vi "Assemble.vi"() -> ()   [LabVIEW 2015]
uses:
  Downloads/fpga_modify-default-myrio-personality/Sub VIs/Utilities/Start Boolean.ctl
  <vilib>/Platform/TimedLoop/XDataNode/timing_clust.ctl
  <vilib>/Platform/TimedLoop/XDataNode/nitl_modes.ctl
  <vilib>/Platform/TimedLoop/XDataNode/wakeup.ctl
  <vilib>/rvi/Emulation/niFpgaGetClockAttributes.vi
  <vilib>/rvi/Emulation/niFpgaSctlEmulationGetInTimedLoop.vi
  <vilib>/rvi/Emulation/niFpgaEmulationReportErrorSimple.vi
  <vilib>/rvi/eio/common/nirviEmuTemplateMethod_errors.vi
  <vilib>/rvi/Emulation/niFpgaCriticalErrorInLSC.vi
  <vilib>/rvi/Emulation/niFpgaProcessEmulError.vi
  <vilib>/rvi/Emulation/niFpgaEmulationIsFPGAContextNoSignature.vi
  <vilib>/rvi/errors/niFpgaSetErrorForExecOnDevCompSimple.vi
  <vilib>/rvi/eio/common/nirviEmuReportErrorAndStop.vi
  <vilib>/rvi/DataTransferAndStorage/Container/Common/niFpgaContainerGetUniqueNameForEmu.vi
  <vilib>/rvi/FIFO/Fifo_Resource/nirvififoEmulationSetSize.vi
  <vilib>/rvi/FIFO/Fifo_Resource/nirviFifoEmulationQueueMgr.vi
  <instcachedir>/0/nirviFifoEmulationQueueMgr_E5CAEC123FF24DC58D834DCA3CDAA9B5.lvgen/nirviFifoEmulationQueueMgr_E5CAEC123FF24DC58D834DCA3CDAA9B5_002.vi
  <vilib>/rvi/FIFO/Fifo_Resource/nirvififoEmulationDetermineInputValidOut.vi
  <vilib>/rvi/FIFO/Fifo_Resource/nirvififoEmulationCreateLock.vi
  <vilib>/rvi/FIFO/Fifo_Resource/nirvififoEmulationObtainLock.vi
  <vilib>/rvi/FIFO/Fifo_Resource/nirvififoEmulationReleaseLock.vi
  <vilib>/rvi/occurrence/nirviWaitOnOccurrenceBase.vi
  <vilib>/rvi/errors/nirviReportUnexpectedCaseInternalError.vi
  <vilib>/rvi/errors/nirviReportUnexpectedCaseInternalError (U32).vi
  <vilib>/Utility/error.llb/Clear Errors.vi
  <vilib>/rvi/DataTransferAndStorage/Container/Common/niFpgaContainerSetEmuInfo.vi
  <vilib>/eio/EIONode/EIONode.xnode
  <vilib>/rvi/DataTransferAndStorage/Container/XNode/niFpgaContainer.xnode
  <vilib>/rvi/FIFO/Fifo_Resource/nirvififoEmulationWrite.vi
  <vilib>/rvi/FIFO/Fifo_Resource/nirvififoEmulationRead.vi
  <vilib>/Platform/TimedLoop/XDataNode/XDataNode.xnode
  <vilib>/rvi/LocalResourceManager/LocalResourceManager.xnode
  <vilib>/rvi/Arithmetic/AddSubMult/XNode/nirviSatArithmetic.xnode
  <vilib>/Platform/TimedLoop/XDataNode/XDNodeRunTimeDep.lvlib
panel:
  out "time of flight 4":u32
  out "time of flight 3":u32
  out "time of flight 2":u32
  out "time of flight 1":u32
  in  "Trigger pulse interval 4":u32=200
  in  "Trigger pulse interval 3":u32=200
  in  "Trigger pulse interva 2":u32=200
  out "Velocity (Counts/Interval) 4":i32
  out "Acceleration (Counts/Interval) 4":i32
  in  "Velocity Interval (uSec) 4":u32=1000
  out "Velocity (Counts/Interval) 3":i32
  out "Acceleration (Counts/Interval) 3":i32
  in  "Velocity Interval (uSec) 3":u32=1000
  out "Velocity (Counts/Interval) 2":i32
  out "Acceleration (Counts/Interval) 2":i32
  in  "Velocity Interval (uSec) 2":u32=1000
  out "Velocity (Counts/Interval)":i32
  out "Acceleration (Counts/Interval)":i32
  in  "Velocity Interval (uSec)":u32=1000
  out "Position 4":i32
  in  "Position Reset 4":bool
  out "Position 3":i32
  in  "Position Reset 3":bool
  in  "En8":bool
  in  "En7":bool
  in  "En6":bool
  in  "En5":bool
  in  "En4":bool
  in  "En3":bool
  in  "En2":bool
  in  "En1":bool
  in  "Relay Motor 1":bool=TRUE
  in  "Relay motor 2":bool=TRUE
  in  "Relay motor 3":bool=TRUE
  in  "Relay motor 4":bool=TRUE
  in  "Relay kebocoran":bool=TRUE
  in  "tof 8":u32=200
  in  "EI8":bool=TRUE
  in  "ton 8":u32=10
  in  "E8O":bool=TRUE
  in  "tof 7":u32=200
  in  "EI7":bool=TRUE
  in  "ton 7":u32=10
  in  "E7O":bool=TRUE
  in  "tof 6":u32=200
  in  "EI6":bool=TRUE
  in  "ton 6":u32=10
  in  "E6O":bool=TRUE
  in  "tof 5":u32=200
  in  "EI54":bool=TRUE
  in  "ton 5":u32=10
  in  "E5O":bool=TRUE
  in  "tof 4":u32=200
  in  "EI4":bool=TRUE
  in  "ton 4":u32=10
  in  "E4O":bool=TRUE
  in  "tof 3":u32=200
  in  "EI3":bool=TRUE
  in  "ton 3":u32=10
  in  "E3O":bool=TRUE
  in  "tof 2":u32=200
  in  "ton 2":u32=10
  in  "EI2":bool=TRUE
  in  "EI1":bool=TRUE
  in  "E2O":bool=TRUE
  in  "E1O":bool=TRUE
  in  "ton":u32=10
  in  "tof":u32=200
  out "Position 2":i32
  in  "Position Reset 2":bool
  in  "Position Reset":bool
  out "Position 1":i32
  in  "I2C.A.DATO 2":u8
  out "I2C.A.DATI 2":u8
  in  "I2C.A.ADDR 2":u8 format="%08.0f"
  in  "I2C.A.CNTR 2":u8=213
  in  "I2C.A.CNTL 2":u8 format="%08b"
  out "I2C.A.STAT 2":u8 format="%08b"
  in  "I2C.A.CNFG 2":u8=1 format="%08b"
  in  "Execute?":T1
  in  "OUT 0":bool
  out "LIMIT BAWAH":bool
  out "LIMIT ATAS":bool
  out "BUTTON":bool
  in  "Trigger pulse interval 1":u32=200
  out "Channel 1":u32
  out "Channel) 2":u32
  out "Channel 3":u32
  in  "IRQ.TIMER.SETTIME":T1
  in  "IRQ.TIMER.WRITE":u32
  out "IRQ.TIMER.READ":u32
  out "ACC.Z.VAL":u16
  out "SYS.ACC.RDY":bool
  out "ACC.Y.VAL":u16
  out "ACC.X.VAL":u16
  in  "DO.LED3:0":u8 format="%04b"
  out "DI.BTN":u8 format="%08b"
  in  "IRQ.DI_BTN.ENA":bool
  in  "IRQ.DI_BTN.RISE":bool
  in  "IRQ.DI_BTN.FALL":bool
  in  "IRQ.DI_BTN.CNT":u32
  in  "IRQ.DI_BTN.NO":u8
  out "SYS.RDY":bool
  out "AI.A_0.VAL":u16
  out "V sensor":u16
  out "Water_LVL1":u16
  out "Water_LVL2":u16
  out "ACS712(1)":u16
  out "ACS712(2)":u16
  out "ACS712(3)":u16
  out "ACS712(4)":u16
  out "SYS.AI.RDY":bool
  out "AI.AudioIn_L.VAL":u16
  out "AI.AudioIn_R.VAL":u16
  out "AI.C_1.VAL":u16
  out "AI.C_0.VAL":u16
  in  "IRQ.AI_A_3:0.CNFG":u8 format="%.0b"
  in  "IRQ.AI_A_0.THRESHOLD":u16
  in  "IRQ.AI_A_1.THRESHOLD":u16
  in  "IRQ.AI_A_0.NO":u8
  in  "IRQ.AI_A_1.NO":u8
  in  "IRQ.AI_A_1.HYSTERESIS":u16=17
  in  "IRQ.AI_A_0.HYSTERESIS":u16=17
  in  "AO.A_0.VAL":u16
  in  "AO.A_1.VAL":u16
  in  "AO.B_0.VAL":u16
  in  "AO.B_1.VAL":u16
  in  "AO.AudioOut_L.VAL":u16
  in  "AO.AudioOut_R.VAL":u16
  in  "AO.SYS.GO":T1
  in  "AO.C_1.VAL":u16
  in  "AO.C_0.VAL":u16
  out "AO.SYS.STAT":bool
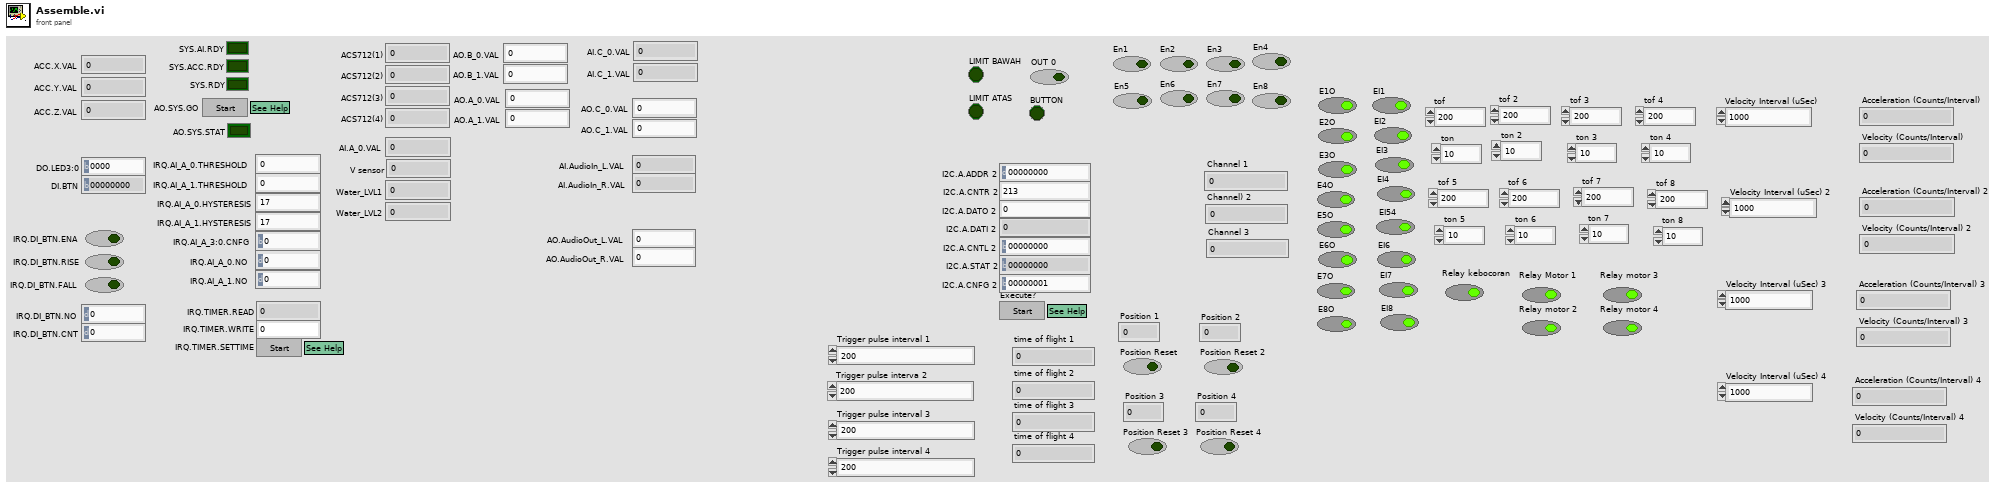
[diagram p1: front panel]
types:
  T1 = typedef "Start Boolean.ctl" = bool
  T2 = typedef "XDNodeRunTimeDep.lvlib/timing_clust.ctl" = cluster{"Expected End [f-1]":u64, "Actual End [f-1]":u64, "Finished Late? [f-1]":bool, "Expected End [i-1]":u64, "Actual End [i-1]":u64, "Finished Late? [i-1]":bool, "Expected Start [i]":u64, "Actual Start [i]":u64, "Expected Start [f]":u64, "Actual Start [f]":u64, "Source Name":string, "Structure Name":string, "Period":i64, "Deadline":i64, "Offset":i64, "Start":i64, "Priority":i32, "Timeout":i32, "Mode":T3, "Wakeup Reason":T4, "Error":errorcluster, "Source Type":string, "Secondary Source Type":string, "Global End Time":u64, "Global Start Time":u64, "Frame Duration":u64, "Iteration Duration":u64, "Assigned CPU":i32, "I/O Scan Engine Mode":u32}
  T3 = typedef "XDNodeRunTimeDep.lvlib/nitl_modes.ctl" = enum32{"No Change", "Process missed periods, maintain original phase", "Discard missed periods, maintain original phase", "Process missed periods, ignore original phase", "Discard missed periods, ignore original phase"}
  T4 = typedef "XDNodeRunTimeDep.lvlib/wakeup.ctl" = enum32{"Normal", "Aborted", "Asynchronous wakeup", "Timing source error", "Timed loop error", "Timeout"}
diagram:
  # "The Timed Loop does not allow writing the same FIFO outside the Timed Loop. Use another FIFO to push all interrupts from Button in the Timed Loop to the IRQ Queue."
  # "The accelerometer nodes take some time before the FPGA can first read the values. This is because it takes time to read from the accelerometer. An iteration of the While Loop will not complete until the accelerometer values have been read.\n\nAfter the completion of the first iteration of the While Loop, all indicators have valid values."
  # "The analog output nodes take some time before the FPGA write the values to the pins. The GO and STAT registers are used to handshake between the FPGA and host. When the host wants the values to be written, the host sets the GO register to TRUE. If the host reads the STAT register before setting the value of the GO register, it can wait for the value of the STAT register to invert. The value inversion tells the host that the output values have been written."
  # "The analog input nodes take some time before the FPGA can first read the values. This is because it takes time to set up the Analog-to-Digital converter (ADC) and convert the first reading. An iteration of the While Loop will not complete until all the analog input channels have been sampled.\n\nAfter the completion of the first iteration of the While Loop, all indicators have valid values."
  # "Note: On some hardware a \"ghosting effect\" may occur on any unconnected AI channels. For example, if channel AI0 is connected and channels AI1~AI7 are not connected the the value read at AI0 may be seen on indicators AI1~AI7. This is common for hardware that use a multiplexed (MUXed) Analog-to-Digital converter (ADC), because the input analog signal is used to charge a capacitor which does not discharge before the unconnected channel is read.\n\nYou can hide the \"ghosting effect\" by using an mask register. This register is used to decide when the indicator should be updated."
  # "The FPGA timer fires the interrupt request (IRQ) when TIMER.Read counts down to zero. If TIMER.Read is not zero, it counts down to one per microsecond."
  # "The only interface that sends interrupts to the RT side. Timer interrupts, analog input interrupts, digital input interrupts, and SPI interrupt share this interface.\n\nAll interrupts work in sequence. One interrupt waits until the previous interrupt request (IRQ) gets acknowledged on the RT side."
  # "NOTE: The SYS.RDY Boolean MUST exist and must become TRUE at some point. Otherwise, the myRIO VIs will not function correctly."
  # "There is some delay between the time when the FPGA code starts and the time when the analog inputs, accelerometer, and scaling values outputs are valid. If the host wants to ensure that there are valid values in theses registers it should wait for each subsystem to finish its initialization process. \n\nWhen all subsystems have finished initializinig, the SYS.RDY indicator turns true. The host can poll the SYS.RDY indicator to determine the status of the FPGA. Alternatively, the host can poll the individual SYS.xx.RDY indicators to determine the status of the individual subsystems.\n\nThis loop continues indefinitely, essentially making SYS.RDY a read-only register."
  n1 = while {
    stop <- FALSE stop-if-true
    # "Host Synchronization"
    n2 = local read "SYS.ACC.RDY"() -> (w24:bool)
    n3 = local read "SYS.AI.RDY"() -> (w26:bool)
    n4 = Compound Arithmetic op=AND(w26, w24) -> (→"SYS.RDY":bool)
  }
  n5 = while {
    stop <- FALSE stop-if-true
    # "Interrupt to RT"
    n6 = xnode ("FIFO Method Node")("Timeout"=-1) -> ("Element"=w29:u8)  [unwired: 1 in, 2 out]
    n7 = call <vilib>:"niFPGA Interrupt.vi"("Wait Until Cleared (F)"=TRUE, "IRQ Number (0)"=w29) -> ()  [unwired: 1 in]
  }
  n8 = while {
    stop <- FALSE stop-if-true
    # "Timer"
    n9 = local read "IRQ.TIMER.READ"() -> (w34:u32)
    n10 = Select(t="IRQ.TIMER.WRITE", s="IRQ.TIMER.SETTIME", f=w34) -> (s? t:f=w32:u32)
    n11 = case shown="Default" w32 {
      selector: w32 -> [w38 w41]
      tunnel: [w38 w39] -> w31
      frame 0 {
      }
      frame Default {
        n12 = Decrement(x=w41) -> (x-1=w40:u32)
        n13 = case shown="0" w40 {
          selector: w40 -> [w42 w45]
          tunnel: [w42 w45] -> w39
          frame Default {
          }
          frame 0 {
            w44 = u8 0  # Reserved for Timer IRQ
            n14 = xnode ("FIFO Method Node")("Element"=w44, "Timeout"=-1) -> ()  [unwired: 1 in, 2 out]
          }
        }
      }
    }
    "IRQ.TIMER.READ" <- w31
    n15 = call "Loop Timer"("Count(uSec)"=u8 1 ("Count(mSec)")) -> ()  [unwired: 1 out]
  }
  n16 = xnode "VI-Defined FIFO Configuration"() -> ("FIFO Out"=w20:refnum<k21>)
  n17 = while {
    tunnel: w20 -> [w47]
    i -> [w74]
    stop <- FALSE stop-if-true
    # "Analog Input"
    n18 = xnode "FPGA I/O Node"() -> ("ConnectorA/AI0"=w52:u16, "ConnectorA/AI1"=w51:u16, "ConnectorA/AI2"=→"Water_LVL1":u16, "ConnectorA/AI3"=→"Water_LVL2":u16, "ConnectorB/AI0"=→"ACS712(1)":u16, "ConnectorB/AI1"=→"ACS712(2)":u16, "ConnectorB/AI2"=→"ACS712(3)":u16, "ConnectorB/AI3"=→"ACS712(4)":u16, "ConnectorC/AI0"=w68:i16, "ConnectorC/AI1"=w67:i16, "AudioIn/Left"=w66:i16, "AudioIn/Right"=w65:i16)  [unwired: 12 in, 12 out]
    "AI.A_0.VAL" <- w52
    "V sensor" <- w51
    n19 = Greater Than 0?(x=w74) -> (x > 0?=→"SYS.AI.RDY":bool)
    n20 = Number To Boolean Array(number="IRQ.AI_A_3:0.CNFG") -> (Boolean array=w62:bool[])
    n21 = Index Array(array=w62) -> (element #1=w60:bool, element #2=w59:bool, element #3=w57:bool, element #4=w56:bool)  [unwired: 4 in]
    n22 = To Unsigned Word Integer(number=w68) -> (unsigned 16bit integer=→"AI.C_0.VAL":u16)
    n23 = To Unsigned Word Integer(number=w67) -> (unsigned 16bit integer=→"AI.C_1.VAL":u16)
    n24 = To Unsigned Word Integer(number=w66) -> (unsigned 16bit integer=→"AI.AudioIn_L.VAL":u16)
    n25 = To Unsigned Word Integer(number=w65) -> (unsigned 16bit integer=→"AI.AudioIn_R.VAL":u16)
    n26 = call "Check AI IRQ.vi"("Hysteresis"="IRQ.AI_A_1.HYSTERESIS", "FIFO In"=w47, "IRQ Number"="IRQ.AI_A_1.NO", "Threshold"="IRQ.AI_A_1.THRESHOLD", "Analog Value"=w51, "Rising Edge?"=w56, "Enable Interrupt?"=w57) -> ()  [unwired: 5 in]
    n27 = call "Check AI IRQ.vi"("Hysteresis"="IRQ.AI_A_0.HYSTERESIS", "FIFO In"=w47, "IRQ Number"="IRQ.AI_A_0.NO", "Threshold"="IRQ.AI_A_0.THRESHOLD", "Analog Value"=w52, "Rising Edge?"=w59, "Enable Interrupt?"=w60) -> ()  [unwired: 5 in]
  }
  n28 = while {
    stop <- FALSE stop-if-true
    # "Analog Output"
    n29 = feedback #1(FALSE) -> (w80:bool)
    n30 = case shown="True" "AO.SYS.GO" {
      tunnel: "AO.C_0.VAL" -> [_ w102]
      tunnel: "AO.C_1.VAL" -> [_ w101]
      tunnel: "AO.A_0.VAL" -> [_ w106]
      tunnel: "AO.A_1.VAL" -> [_ w105]
      tunnel: "AO.B_0.VAL" -> [_ w104]
      tunnel: "AO.B_1.VAL" -> [_ w103]
      tunnel: "AO.AudioOut_L.VAL" -> [_ w98]
      tunnel: "AO.AudioOut_R.VAL" -> [_ w97]
      tunnel: w80 -> [w91 w94]
      tunnel: [w91 w92] -> w78
      frame False {
      }
      frame True {
        n31 = To Word Integer(number=w102) -> (16bit integer=w100:i16)
        n32 = To Word Integer(number=w101) -> (16bit integer=w99:i16)
        n33 = To Word Integer(number=w98) -> (16bit integer=w96:i16)
        n34 = To Word Integer(number=w97) -> (16bit integer=w95:i16)
        n35 = flat-sequence {
          tunnel: w106 -> [w115]
          tunnel: w105 -> [w114]
          tunnel: w104 -> [w113]
          tunnel: w103 -> [w112]
          tunnel: w100 -> [w111]
          tunnel: w99 -> [w110]
          tunnel: w96 -> [w109]
          tunnel: w95 -> [w108]
          tunnel: w94 -> [w107]
          tunnel: [w107] -> w93
          tunnel: w93 -> [w117]
          tunnel: [w116] -> w92
          frame #0 {
            n36 = xnode "FPGA I/O Node"("ConnectorA/AO0"=w115, "ConnectorA/AO1"=w114, "ConnectorB/AO0"=w113, "ConnectorB/AO1"=w112, "ConnectorC/AO0"=w111, "ConnectorC/AO1"=w110, "AudioOut/Left"=w109, "AudioOut/Right"=w108) -> ()  [unwired: 8 in, 8 out]
          }
          frame #1 {
            n37 = Not(x=w117) -> (.not. x?=w116:bool)
          }
        }
      }
    }
    "AO.SYS.STAT" <- w78
    n38 = feedback-in #1(w78) -> ()
  }
  n39 = while {
    i -> [w122]
    stop <- FALSE stop-if-true
    # "Onboard Accelerometer"
    n40 = xnode "FPGA I/O Node"() -> ("AccelerationX"=w125:i16, "AccelerationY"=w124:i16, "AccelerationZ"=w123:i16)  [unwired: 3 in, 3 out]
    n41 = Greater Than 0?(x=w122) -> (x > 0?=→"SYS.ACC.RDY":bool)
    n42 = To Unsigned Word Integer(number=w125) -> (unsigned 16bit integer=→"ACC.X.VAL":u16)
    n43 = To Unsigned Word Integer(number=w124) -> (unsigned 16bit integer=→"ACC.Y.VAL":u16)
    n44 = To Unsigned Word Integer(number=w123) -> (unsigned 16bit integer=→"ACC.Z.VAL":u16)
  }
  n45 = xnode "VI-Defined FIFO Configuration"() -> ("FIFO Out"=w19:refnum<k21>)
  n46 = node-c288() -> (w22:T2)  [unwired: 1 in]
  n47 = timed-loop {
    timing: w22 -> [_]
    timing-out: [_] -> w21
    tunnel: w19 -> [w129]
    stop <- _ stop-if-true
    # "Onboard DIO"
    n48 = xnode "FPGA I/O Node"() -> ("Button0"=w133:bool)  [unwired: 1 in, 1 out]
    n49 = Number To Boolean Array(number="DO.LED3:0") -> (Boolean array=w138:bool[])
    n50 = Build Array(w133) -> (w141:bool[])
    n51 = Index Array(array=w138) -> (element #1=w137:bool, element #2=w136:bool, element #3=w135:bool, element #4=w134:bool)  [unwired: 4 in]
    n52 = call "DIO IRQ 1-bit.vi"("IRQ.NO"="IRQ.DI_BTN.NO", "IRQ.CNT"="IRQ.DI_BTN.CNT", "FIFO in"=w129, "IRQ.FALL"="IRQ.DI_BTN.FALL", "IRQ.RISE"="IRQ.DI_BTN.RISE", "IRQ.ENA"="IRQ.DI_BTN.ENA", "DIO"=w133) -> ()  [unwired: 5 in]
    n53 = Boolean Array To Number(Boolean array=w141) -> (number=→"DI.BTN":u8)
    n54 = xnode "FPGA I/O Node"("LED0"=w137, "LED1"=w136, "LED2"=w135, "LED3"=w134) -> ()  [unwired: 4 in, 4 out]
  }
  n55 = while {
    stop <- FALSE stop-if-true
    # "Button SCTL Interrupt Buffer"
    n56 = feedback #2(u8 0 ("Element")) -> (w146:u8)
    n57 = feedback #3(FALSE ("Timed Out?")) -> (w150:bool)
    n58 = case shown="False" w150 {
      tunnel: [w152 w154] -> w147
      tunnel: w146 -> [_ w154]
      frame False {
        n59 = xnode ("FIFO Method Node")("Timeout"=-1) -> ("Element"=w152:u8)  [unwired: 1 in, 2 out]
      }
      frame True {
      }
    }
    n60 = feedback-in #2(w147) -> ()
    n61 = xnode ("FIFO Method Node")("Element"=w147, "Timeout"=0) -> ("Timed Out?"=w148:bool)  [unwired: 1 in, 1 out]
    n62 = feedback-in #3(w148) -> ()
  }
  n63 = node-c288(w21) -> ()
  n64 = node-c288() -> (w16:T2)  [unwired: 1 in]
  n65 = timed-loop {
    timing: w16 -> [_]
    timing-out: [_] -> w15
    stop <- _ stop-if-true
    # "Connector ALL DIO"
    n66 = disable-structure shown="Disabled" {
      frame Disabled {
        # "DIGITAL BUTTON LAMP"
        # "LIMIT"
        # "I2C MASTER"
        n67 = call "DIO 1-bit.vi"("DIR"=FALSE, "DIO Refnum"=refnum<k21> "ConnectorB/DIO15") -> ("IN"=→"LIMIT ATAS":bool)  [unwired: 9 in]
        n68 = call "DIO 1-bit.vi"("DIR"=FALSE, "DIO Refnum"=refnum<k21> "ConnectorB/DIO14") -> ("IN"=→"LIMIT BAWAH":bool)  [unwired: 9 in]
        n69 = call "DIO 1-bit.vi"("DIR"=TRUE, "OUT"="OUT 0", "DIO Refnum"=refnum<k21> "ConnectorB/DIO15") -> ()  [unwired: 8 in, 1 out]
        n70 = call "DIO 1-bit.vi"("DIR"=FALSE, "DIO Refnum"=refnum<k21> "ConnectorB/DIO14") -> ("IN"=w156:bool)  [unwired: 9 in]
        n71 = call "DIO_I2C.vi"("I2C.CNFG"="I2C.A.CNFG 2", "I2C.CNTL"="I2C.A.CNTL 2", "I2C.ADDR"="I2C.A.ADDR 2", "I2C.DATO"="I2C.A.DATO 2", "DIO.1/I2C.SDA"=refnum<k21> "ConnectorA/DIO15" ("DIO.1/I2C.SCL"), "I2C.CNTR"="I2C.A.CNTR 2", "DIO.0/I2C.SCL"=refnum<k21> "ConnectorA/DIO14" ("DIO.0/I2C.SDA"), "Execute?"="Execute?", "SELECT"=TRUE) -> ("I2C.DATI"=→"I2C.A.DATI 2":u8, "I2C.STAT"=→"I2C.A.STAT 2":u8)  [unwired: 8 in, 1 out]
        n72 = Not(x=w156) -> (.not. x?=→"BUTTON":bool)
      }
      frame Enabled {
      }
    }
  }
  n73 = node-c288(w15) -> ()
  n74 = node-c288() -> (w2:T2)  [unwired: 1 in]
  n75 = node-c288() -> (w4:T2)  [unwired: 1 in]
  n76 = node-c288() -> (w6:T2)  [unwired: 1 in]
  n77 = node-c288() -> (w8:T2)  [unwired: 1 in]
  n78 = timed-loop "Pulsewidth Measurement + Sound Output" {
    shift-left: _ -> [w190]
    shift-right: [w183] -> _
    shift-left: _ -> [w189]
    shift-right: [w188] -> _
    shift-left: _ -> [w186]
    shift-right: [w184] -> _
    timing: w2 -> [_]
    timing-out: [_] -> w1
    stop <- FALSE stop-if-true
    # "Ultrasonic Echo"
    n79 = call "Count4"() -> ("Tick Count(uSec)"=w181:u32)
    n80 = xnode "FPGA I/O Node"() -> ("ConnectorA/DIO7"=w184:bool)  [unwired: 1 in, 1 out]
    n81 = Greater?(x=w184, y=w186) -> (0:w187:bool)
    n82 = Less?(x=w184, y=w186) -> (x < y?=w185:bool)
    n83 = Select(t=w181, s=w187, f=w189) -> (s? t:f=w188:u32)
    n84 = case shown="True" w185 {
      tunnel: w190 -> [_ w194]
      tunnel: w181 -> [w191 _]
      tunnel: w189 -> [w192 _]
      tunnel: [w193 w194] -> w183
      frame True {
        n85 = Subtract(x=w191, y=w192) -> (x-y=w193:u32)
      }
      frame False {
      }
    }
    "time of flight 4" <- w183
  }
  n86 = timed-loop "Pulsewidth Measurement + Sound Output" {
    shift-left: _ -> [w206]
    shift-right: [w199] -> _
    shift-left: _ -> [w205]
    shift-right: [w204] -> _
    shift-left: _ -> [w202]
    shift-right: [w200] -> _
    timing: w4 -> [_]
    timing-out: [_] -> w3
    stop <- FALSE stop-if-true
    # "Ultrasonic Echo"
    n87 = call "Count3"() -> ("Tick Count(uSec)"=w197:u32)
    n88 = xnode "FPGA I/O Node"() -> ("ConnectorA/DIO5"=w200:bool)  [unwired: 1 in, 1 out]
    n89 = Greater?(x=w200, y=w202) -> (0:w203:bool)
    n90 = Less?(x=w200, y=w202) -> (x < y?=w201:bool)
    n91 = Select(t=w197, s=w203, f=w205) -> (s? t:f=w204:u32)
    n92 = case shown="True" w201 {
      tunnel: w206 -> [_ w210]
      tunnel: w197 -> [w207 _]
      tunnel: w205 -> [w208 _]
      tunnel: [w209 w210] -> w199
      frame True {
        n93 = Subtract(x=w207, y=w208) -> (x-y=w209:u32)
      }
      frame False {
      }
    }
    "time of flight 3" <- w199
  }
  n94 = timed-loop "Pulsewidth Measurement + Sound Output" {
    shift-left: _ -> [w222]
    shift-right: [w215] -> _
    shift-left: _ -> [w221]
    shift-right: [w220] -> _
    shift-left: _ -> [w218]
    shift-right: [w216] -> _
    timing: w6 -> [_]
    timing-out: [_] -> w5
    stop <- FALSE stop-if-true
    # "Ultrasonic Echo"
    n95 = call "Count2"() -> ("Tick Count(uSec)"=w213:u32)
    n96 = xnode "FPGA I/O Node"() -> ("ConnectorA/DIO3"=w216:bool)  [unwired: 1 in, 1 out]
    n97 = Greater?(x=w216, y=w218) -> (0:w219:bool)
    n98 = Less?(x=w216, y=w218) -> (x < y?=w217:bool)
    n99 = Select(t=w213, s=w219, f=w221) -> (s? t:f=w220:u32)
    n100 = case shown="True" w217 {
      tunnel: w222 -> [_ w226]
      tunnel: w213 -> [w223 _]
      tunnel: w221 -> [w224 _]
      tunnel: [w225 w226] -> w215
      frame True {
        n101 = Subtract(x=w223, y=w224) -> (x-y=w225:u32)
      }
      frame False {
      }
    }
    "time of flight 2" <- w215
  }
  n102 = timed-loop "Pulsewidth Measurement + Sound Output" {
    shift-left: _ -> [w238]
    shift-right: [w231] -> _
    shift-left: _ -> [w237]
    shift-right: [w236] -> _
    shift-left: _ -> [w234]
    shift-right: [w232] -> _
    timing: w8 -> [_]
    timing-out: [_] -> w7
    stop <- FALSE stop-if-true
    # "Ultrasonic Echo"
    n103 = call "Count"() -> ("Tick Count(uSec)"=w229:u32)
    n104 = xnode "FPGA I/O Node"() -> ("ConnectorA/DIO1"=w232:bool)  [unwired: 1 in, 1 out]
    n105 = Greater?(x=w232, y=w234) -> (0:w235:bool)
    n106 = Less?(x=w232, y=w234) -> (x < y?=w233:bool)
    n107 = Select(t=w229, s=w235, f=w237) -> (s? t:f=w236:u32)
    n108 = case shown="True" w233 {
      tunnel: w238 -> [_ w242]
      tunnel: w229 -> [w239 _]
      tunnel: w237 -> [w240 _]
      tunnel: [w241 w242] -> w231
      frame True {
        n109 = Subtract(x=w239, y=w240) -> (x-y=w241:u32)
      }
      frame False {
      }
    }
    "time of flight 1" <- w231
  }
  n110 = while {
    stop <- FALSE stop-if-true
    # "PWM MOTOR"
    n111 = flat-sequence {
      frame #0 {
        n112 = xnode "FPGA I/O Node"("ConnectorB/DIO8"="E1O") -> ()  [unwired: 1 in, 1 out]
      }
      frame #1 {
        n113 = call "Wait3"("Count(uSec)"="ton") -> ()  [unwired: 1 out]
      }
      frame #2 {
        n114 = xnode "FPGA I/O Node"("ConnectorB/DIO8"="EI1") -> ()  [unwired: 1 in, 1 out]
      }
      frame #3 {
        n115 = call "Wait4"("Count(uSec)"="tof") -> ()  [unwired: 1 out]
      }
    }
    n116 = flat-sequence {
      frame #0 {
        n117 = xnode "FPGA I/O Node"("ConnectorB/DIO10"="E3O") -> ()  [unwired: 1 in, 1 out]
      }
      frame #1 {
        n118 = call "Wait7"("Count(uSec)"="ton 3") -> ()  [unwired: 1 out]
      }
      frame #2 {
        n119 = xnode "FPGA I/O Node"("ConnectorB/DIO10"="EI3") -> ()  [unwired: 1 in, 1 out]
      }
      frame #3 {
        n120 = call "Wait8"("Count(uSec)"="tof 3") -> ()  [unwired: 1 out]
      }
    }
    n121 = flat-sequence {
      frame #0 {
        n122 = xnode "FPGA I/O Node"("ConnectorB/DIO9"="E2O") -> ()  [unwired: 1 in, 1 out]
      }
      frame #1 {
        n123 = call "Wait5"("Count(uSec)"="ton 2") -> ()  [unwired: 1 out]
      }
      frame #2 {
        n124 = xnode "FPGA I/O Node"("ConnectorB/DIO9"="EI2") -> ()  [unwired: 1 in, 1 out]
      }
      frame #3 {
        n125 = call "Wait6"("Count(uSec)"="tof 2") -> ()  [unwired: 1 out]
      }
    }
    n126 = flat-sequence {
      frame #0 {
        n127 = xnode "FPGA I/O Node"("ConnectorA/DIO8"="E4O") -> ()  [unwired: 1 in, 1 out]
      }
      frame #1 {
        n128 = call "Wait9"("Count(uSec)"="ton 4") -> ()  [unwired: 1 out]
      }
      frame #2 {
        n129 = xnode "FPGA I/O Node"("ConnectorA/DIO8"="EI4") -> ()  [unwired: 1 in, 1 out]
      }
      frame #3 {
        n130 = call "Wait10"("Count(uSec)"="tof 4") -> ()  [unwired: 1 out]
      }
    }
    n131 = flat-sequence {
      frame #0 {
        n132 = xnode "FPGA I/O Node"("ConnectorA/DIO9"="E5O") -> ()  [unwired: 1 in, 1 out]
      }
      frame #1 {
        n133 = call "Wait11"("Count(uSec)"="ton 5") -> ()  [unwired: 1 out]
      }
      frame #2 {
        n134 = xnode "FPGA I/O Node"("ConnectorA/DIO8"="EI54") -> ()  [unwired: 1 in, 1 out]
      }
      frame #3 {
        n135 = call "Wait12"("Count(uSec)"="tof 5") -> ()  [unwired: 1 out]
      }
    }
    n136 = flat-sequence {
      frame #0 {
        n137 = xnode "FPGA I/O Node"("ConnectorA/DIO10"="E6O") -> ()  [unwired: 1 in, 1 out]
      }
      frame #1 {
        n138 = call "Wait13"("Count(uSec)"="ton 6") -> ()  [unwired: 1 out]
      }
      frame #2 {
        n139 = xnode "FPGA I/O Node"("ConnectorA/DIO10"="EI6") -> ()  [unwired: 1 in, 1 out]
      }
      frame #3 {
        n140 = call "Wait14"("Count(uSec)"="tof 6") -> ()  [unwired: 1 out]
      }
    }
    n141 = flat-sequence {
      frame #0 {
        n142 = xnode "FPGA I/O Node"("ConnectorC/DIO7"="E8O") -> ()  [unwired: 1 in, 1 out]
      }
      frame #1 {
        n143 = call "Wait17"("Count(uSec)"="ton 8") -> ()  [unwired: 1 out]
      }
      frame #2 {
        n144 = xnode "FPGA I/O Node"("ConnectorC/DIO7"="EI8") -> ()  [unwired: 1 in, 1 out]
      }
      frame #3 {
        n145 = call "Wait18"("Count(uSec)"="tof 8") -> ()  [unwired: 1 out]
      }
    }
    n146 = flat-sequence {
      frame #0 {
        n147 = xnode "FPGA I/O Node"("ConnectorC/DIO3"="E7O") -> ()  [unwired: 1 in, 1 out]
      }
      frame #1 {
        n148 = call "Wait15"("Count(uSec)"="ton 7") -> ()  [unwired: 1 out]
      }
      frame #2 {
        n149 = xnode "FPGA I/O Node"("ConnectorC/DIO3"="EI7") -> ()  [unwired: 1 in, 1 out]
      }
      frame #3 {
        n150 = call "Wait16"("Count(uSec)"="tof 7") -> ()  [unwired: 1 out]
      }
    }
  }
  n151 = while {
    stop <- FALSE stop-if-true
    # "Trigger Ultrasonic"
    n152 = flat-sequence {
      frame #0 {
        n153 = xnode "FPGA I/O Node"("ConnectorA/DIO2"=TRUE ("ConnectorC/DIO6")) -> ()  [unwired: 1 in, 1 out]
      }
      frame #1 {
        n154 = call "Wait19"("Count(uSec)"=u32 10) -> ()  [unwired: 1 out]
      }
      frame #2 {
        n155 = xnode "FPGA I/O Node"("ConnectorA/DIO2"=FALSE ("ConnectorC/DIO6")) -> ()  [unwired: 1 in, 1 out]
      }
      frame #3 {
        n156 = call "Wait20"("Count(uSec)"="Trigger pulse interva 2") -> ()  [unwired: 1 out]
      }
    }
    n157 = flat-sequence {
      frame #0 {
        n158 = xnode "FPGA I/O Node"("ConnectorA/DIO0"=TRUE ("ConnectorC/DIO6")) -> ()  [unwired: 1 in, 1 out]
      }
      frame #1 {
        n159 = call "Wait"("Count(uSec)"=u32 10) -> ()  [unwired: 1 out]
      }
      frame #2 {
        n160 = xnode "FPGA I/O Node"("ConnectorA/DIO0"=FALSE ("ConnectorC/DIO6")) -> ()  [unwired: 1 in, 1 out]
      }
      frame #3 {
        n161 = call "Wait2"("Count(uSec)"="Trigger pulse interval 1") -> ()  [unwired: 1 out]
      }
    }
    n162 = flat-sequence {
      frame #0 {
        n163 = xnode "FPGA I/O Node"("ConnectorA/DIO4"=TRUE ("ConnectorC/DIO6")) -> ()  [unwired: 1 in, 1 out]
      }
      frame #1 {
        n164 = call "Wait21"("Count(uSec)"=u32 10) -> ()  [unwired: 1 out]
      }
      frame #2 {
        n165 = xnode "FPGA I/O Node"("ConnectorA/DIO4"=FALSE ("ConnectorC/DIO6")) -> ()  [unwired: 1 in, 1 out]
      }
      frame #3 {
        n166 = call "Wait22"("Count(uSec)"="Trigger pulse interval 3") -> ()  [unwired: 1 out]
      }
    }
    n167 = flat-sequence {
      frame #0 {
        n168 = xnode "FPGA I/O Node"("ConnectorA/DIO6"=TRUE ("ConnectorC/DIO6")) -> ()  [unwired: 1 in, 1 out]
      }
      frame #1 {
        n169 = call "Wait23"("Count(uSec)"=u32 10) -> ()  [unwired: 1 out]
      }
      frame #2 {
        n170 = xnode "FPGA I/O Node"("ConnectorA/DIO6"=FALSE ("ConnectorC/DIO6")) -> ()  [unwired: 1 in, 1 out]
      }
      frame #3 {
        n171 = call "Wait24"("Count(uSec)"="Trigger pulse interval 4") -> ()  [unwired: 1 out]
      }
    }
  }
  n172 = node-c288(w1) -> ()
  n173 = node-c288(w3) -> ()
  n174 = node-c288(w5) -> ()
  n175 = node-c288(w7) -> ()
  n176 = node-c288() -> (w18:T2)  [unwired: 1 in]
  n177 = node-c288() -> (w14:T2)  [unwired: 1 in]
  n178 = timed-loop "Pulsewidth Measurement + Sound Output" {
    shift-left: _ -> [w319]
    shift-right: [w299] -> _
    shift-left: _ -> [w318]
    shift-right: [w298] -> _
    shift-left: _ -> [w316]
    shift-right: [w314] -> _
    shift-right: [w297] -> _
    shift-left: _ -> [w310]
    shift-right: [w300] -> _
    shift-left: _ -> [w309]
    shift-right: [w311] -> _
    shift-left: _ -> [w308]
    shift-right: [w296] -> _
    shift-left: _ -> [w304]
    shift-right: [w301] -> _
    shift-left: _ -> [w303]
    shift-right: [w305] -> _
    shift-left: _ -> [w302]
    timing: w18 -> [_]
    timing-out: [_] -> w17
    stop <- _ stop-if-true
    # "Remote Read"
    n179 = call "Tick Count"() -> ("Tick Count(uSec)"=w295:u32)
    n180 = xnode "FPGA I/O Node"() -> ("ConnectorB/DIO1"=w311:bool)  [unwired: 1 in, 1 out]
    n181 = xnode "FPGA I/O Node"() -> ("ConnectorB/DIO0"=w314:bool)  [unwired: 1 in, 1 out]
    n182 = xnode "FPGA I/O Node"() -> ("ConnectorB/DIO2"=w305:bool)  [unwired: 1 in, 1 out]
    n183 = Greater?(x=w311, y=w308) -> (0:w313:bool)
    n184 = Less?(x=w311, y=w308) -> (x < y?=w312:bool)
    n185 = Greater?(x=w314, y=w316) -> (0:w317:bool)
    n186 = Less?(x=w314, y=w316) -> (x < y?=w315:bool)
    n187 = Greater?(x=w305, y=w302) -> (0:w307:bool)
    n188 = Less?(x=w305, y=w302) -> (x < y?=w306:bool)
    n189 = Select(t=w295, s=w313, f=w310) -> (s? t:f=w297:u32)
    n190 = case shown="True" w312 {
      tunnel: w309 -> [_ w327]
      tunnel: w295 -> [w324 _]
      tunnel: w310 -> [w325 _]
      tunnel: [w326 w327] -> w300
      frame True {
        n191 = Subtract(x=w324, y=w325) -> (x-y=w326:u32)
      }
      frame False {
      }
    }
    "Channel) 2" <- w300
    n192 = Select(t=w295, s=w317, f=w318) -> (s? t:f=w298:u32)
    n193 = case shown="True" w315 {
      tunnel: w319 -> [_ w331]
      tunnel: w295 -> [w328 _]
      tunnel: w318 -> [w329 _]
      tunnel: [w330 w331] -> w299
      frame True {
        n194 = Subtract(x=w328, y=w329) -> (x-y=w330:u32)
      }
      frame False {
      }
    }
    "Channel 1" <- w299
    n195 = Select(t=w295, s=w307, f=w304) -> (s? t:f=w296:u32)
    n196 = case shown="True" w306 {
      tunnel: w303 -> [_ w323]
      tunnel: w295 -> [w320 _]
      tunnel: w304 -> [w321 _]
      tunnel: [w322 w323] -> w301
      frame True {
        n197 = Subtract(x=w320, y=w321) -> (x-y=w322:u32)
      }
      frame False {
      }
    }
    "Channel 3" <- w301
  }
  n198 = timed-loop "32 bit, quadrature counter" {
    shift-right: [w439] -> _
    shift-left: _ -> [w435]
    shift-right: [w374] -> _
    shift-left: _ -> [w436]
    shift-right: [w438] -> _
    shift-left: _ -> [w440]
    timing: w14 -> [_]
    timing-out: [_] -> w13
    shift-right: [w420] -> _
    shift-left: _ -> [w421]
    shift-right: [w419] -> _
    shift-left: _ -> [w422]
    shift-right: [w361] -> _
    shift-left: _ -> [w423]
    shift-right: [w404] -> _
    shift-left: _ -> [w405]
    shift-right: [w403] -> _
    shift-left: _ -> [w406]
    shift-right: [w350] -> _
    shift-left: _ -> [w407]
    shift-right: [w388] -> _
    shift-left: _ -> [w389]
    shift-right: [w387] -> _
    shift-left: _ -> [w390]
    shift-right: [w334] -> _
    shift-left: _ -> [w391]
    shift-right: [w383] -> _
    shift-left: _ -> [w384]
    shift-right: [w382] -> _
    shift-left: _ -> [w380]
    shift-right: [w381] -> _
    shift-left: _ -> [w379]
    shift-right: [w375] -> _
    shift-left: _ -> [w377]
    shift-right: [w376] -> _
    shift-left: _ -> [w378]
    shift-right: [w366] -> _
    shift-left: _ -> [w367]
    shift-right: [w365] -> _
    shift-left: _ -> [w368]
    shift-right: [w364] -> _
    shift-left: _ -> [w369]
    shift-right: [w363] -> _
    shift-left: _ -> [w370]
    shift-right: [w362] -> _
    shift-left: _ -> [w371]
    shift-right: [w351] -> _
    shift-left: _ -> [w348]
    shift-right: [w352] -> _
    shift-left: _ -> [w349]
    shift-right: [w353] -> _
    shift-left: _ -> [w356]
    shift-right: [w354] -> _
    shift-left: _ -> [w357]
    shift-right: [w355] -> _
    shift-left: _ -> [w358]
    shift-right: [w339] -> _
    shift-left: _ -> [w340]
    shift-right: [w338] -> _
    shift-left: _ -> [w341]
    shift-right: [w337] -> _
    shift-left: _ -> [w342]
    shift-right: [w336] -> _
    shift-left: _ -> [w343]
    shift-right: [w335] -> _
    shift-left: _ -> [w344]
    stop <- _ stop-if-true
    # ">>Acceleration (last)>>"
    # "Start Time"
    # ">>    Velocity (last)    >>"
    # ">>   Position (last)   >>"
    # "Time Now"
    # ">>Time Elapsed>>"
    # ">>Acceleration (last)>>"
    # "Start Time"
    # ">>    Velocity (last)    >>"
    # ">>   Position (last)   >>"
    # "Time Now"
    # ">>Time Elapsed>>"
    # ">>Acceleration (last)>>"
    # "Start Time"
    # ">>    Velocity (last)    >>"
    # ">>   Position (last)   >>"
    # "Time Now"
    # ">>Time Elapsed>>"
    # ">>Acceleration (last)>>"
    # "Start Time"
    # ">>    Velocity (last)    >>"
    # ">>   Position (last)   >>"
    # "Time Now"
    # ">>Time Elapsed>>"
    # "A  -> Current Quadrature Encoder Channel A value\nA' -> Last value of Quadrature Encoder Channel A\nB  -> Current Quadrature Encoder Channel B value\nB' -> Last value of Quadrature Encoder Channel B"
    # "A'"
    # "B"
    # "A'"
    # "A"
    # "B'"
    # "B"
    # ">>ChB>>"
    # ">>ChA>>"
    # "A  -> Current Quadrature Encoder Channel A value\nA' -> Last value of Quadrature Encoder Channel A\nB  -> Current Quadrature Encoder Channel B value\nB' -> Last value of Quadrature Encoder Channel B"
    # "A'"
    # "B"
    # "A'"
    # "A"
    # "B'"
    # "B"
    # ">>ChB>>"
    # ">>ChA>>"
    # "A  -> Current Quadrature Encoder Channel A value\nA' -> Last value of Quadrature Encoder Channel A\nB  -> Current Quadrature Encoder Channel B value\nB' -> Last value of Quadrature Encoder Channel B"
    # "A'"
    # "B"
    # "A'"
    # "A"
    # "B'"
    # "B"
    # ">>ChB>>"
    # ">>ChA>>"
    # "A  -> Current Quadrature Encoder Channel A value\nA' -> Last value of Quadrature Encoder Channel A\nB  -> Current Quadrature Encoder Channel B value\nB' -> Last value of Quadrature Encoder Channel B"
    # "A'"
    # "B"
    # "A'"
    # "A"
    # "B'"
    # "B"
    # ">>ChB>>"
    # ">>ChA>>"
    # "Quadrature Encoder"
    n199 = call "Tick Count"() -> ("Tick Count(uSec)"=w345:u32)
    n200 = xnode "FPGA I/O Node"() -> ("ConnectorC/DIO5"=w388:bool, "ConnectorC/DIO6"=w387:bool)  [unwired: 2 in, 2 out]
    n201 = xnode "FPGA I/O Node"() -> ("ConnectorC/DIO2"=w404:bool, "ConnectorC/DIO4"=w403:bool)  [unwired: 2 in, 2 out]
    n202 = xnode "FPGA I/O Node"() -> ("ConnectorB/DIO11"=w439:bool, "ConnectorB/DIO12"=w438:bool)  [unwired: 2 in, 2 out]
    n203 = xnode "FPGA I/O Node"() -> ("ConnectorA/DIO11"=w420:bool, "ConnectorA/DIO12"=w419:bool)  [unwired: 2 in, 2 out]
    n204 = Select(t=w345, s=w384, f=w380) -> (s? t:f=w382:u32)
    n205 = xnode ("Saturation Subtract2")("x"=w345, "y"=w382) -> ("x-y"=w385:u32)
    n206 = Exclusive Or(1:w390, 2:w388) -> (0:w393:bool)
    n207 = Exclusive Or(1:w406, 2:w404) -> (0:w409:bool)
    n208 = Exclusive Or(1:w440, 2:w439) -> (0:w441:bool)
    n209 = Exclusive Or(1:w422, 2:w420) -> (0:w425:bool)
    n210 = Exclusive Or(1:w390, 2:w387) -> (0:w395:bool)
    n211 = Exclusive Or(1:w389, 2:w388) -> (0:w394:bool)
    n212 = Exclusive Or(1:w406, 2:w403) -> (0:w411:bool)
    n213 = Select(t=0 ("32 bit"), s="Position Reset 4", f=w391) -> (s? t:f=w400:i32)
    n214 = Exclusive Or(1:w440, 2:w438) -> (0:w443:bool)
    n215 = Exclusive Or(1:w405, 2:w404) -> (0:w410:bool)
    n216 = Exclusive Or(1:w422, 2:w419) -> (0:w427:bool)
    n217 = Exclusive Or(1:w435, 2:w439) -> (0:w442:bool)
    n218 = Select(t=0 ("32 bit"), s="Position Reset 3", f=w407) -> (s? t:f=w416:i32)
    n219 = Exclusive Or(1:w421, 2:w420) -> (0:w426:bool)
    n220 = Select(t=0 ("32 bit"), s="Position Reset", f=w436) -> (s? t:f=w448:i32)
    n221 = Select(t=0 ("32 bit"), s="Position Reset 2", f=w423) -> (s? t:f=w432:i32)
    n222 = Select(t=w345, s=w367, f=w368) -> (s? t:f=w365:u32)
    n223 = Select(t=-1 ("32 bit"), s=w393, f=1 ("32 bit")) -> (s? t:f=w398:i32)
    n224 = Select(t=-1 ("32 bit"), s=w409, f=1 ("32 bit")) -> (s? t:f=w414:i32)
    n225 = Select(t=-1 ("32 bit"), s=w441, f=1 ("32 bit")) -> (s? t:f=w446:i32)
    n226 = Select(t=-1 ("32 bit"), s=w425, f=1 ("32 bit")) -> (s? t:f=w430:i32)
    n227 = Or(x=w394, y=w395) -> (x .or. y?=w392:bool)
    n228 = Or(x=w410, y=w411) -> (x .or. y?=w408:bool)
    n229 = Select(t=w345, s=w348, f=w349) -> (s? t:f=w352:u32)
    n230 = Or(x=w442, y=w443) -> (x .or. y?=w437:bool)
    n231 = Select(t=w345, s=w340, f=w341) -> (s? t:f=w338:u32)
    n232 = Or(x=w426, y=w427) -> (x .or. y?=w424:bool)
    n233 = xnode ("Saturation Subtract2")("x"=w345, "y"=w365) -> ("x-y"=w372:u32)
    n234 = Add(x=w398, y=w400) -> (x+y=w402:i32)
    n235 = Add(x=w414, y=w416) -> (x+y=w418:i32)
    n236 = Add(x=w446, y=w448) -> (x+y=w450:i32)
    n237 = Add(x=w430, y=w432) -> (x+y=w434:i32)
    n238 = xnode ("Saturation Subtract2")("x"=w345, "y"=w352) -> ("x-y"=w359:u32)
    n239 = xnode ("Saturation Subtract2")("x"=w345, "y"=w338) -> ("x-y"=w346:u32)
    n240 = Greater Or Equal?(x=w385, y="Velocity Interval (uSec)") -> (x >= y?=w383:bool)
    n241 = Select(t=w402, s=w392, f=w400) -> (s? t:f=w334:i32)
    "Position 4" <- w334
    n242 = Select(t=w418, s=w408, f=w416) -> (s? t:f=w350:i32)
    "Position 3" <- w350
    n243 = Select(t=w450, s=w437, f=w448) -> (s? t:f=w374:i32)
    "Position 1" <- w374
    n244 = Select(t=w434, s=w424, f=w432) -> (s? t:f=w361:i32)
    "Position 2" <- w361
    n245 = Greater Or Equal?(x=w372, y="Velocity Interval (uSec) 2") -> (x >= y?=w366:bool)
    n246 = case shown="True" w383 {
      tunnel: w374 -> [_ w626]
      tunnel: w379 -> [w623 w630]
      tunnel: [w625 w629] -> w376
      tunnel: w378 -> [w625 w628]
      tunnel: [w624 w627] -> w375
      tunnel: w377 -> [w624 _]
      tunnel: [w623 w626] -> w381
      frame False {
      }
      frame True {
        n247 = xnode ("Saturation Subtract")("x"=w626, "y"=w630) -> ("x-y"=w629:i32)
        n248 = xnode ("Saturation Subtract3")("x"=w629, "y"=w628) -> ("x-y"=w627:i32)
      }
    }
    "Acceleration (Counts/Interval)" <- w375
    "Velocity (Counts/Interval)" <- w376
    n249 = Greater Or Equal?(x=w359, y="Velocity Interval (uSec) 3") -> (x >= y?=w351:bool)
    n250 = Greater Or Equal?(x=w346, y="Velocity Interval (uSec) 4") -> (x >= y?=w339:bool)
    n251 = case shown="True" w366 {
      tunnel: w361 -> [_ w572]
      tunnel: w369 -> [w569 w576]
      tunnel: [w571 w575] -> w362
      tunnel: w371 -> [w571 w574]
      tunnel: [w570 w573] -> w363
      tunnel: w370 -> [w570 _]
      tunnel: [w569 w572] -> w364
      frame False {
      }
      frame True {
        n252 = xnode ("Saturation Subtract")("x"=w572, "y"=w576) -> ("x-y"=w575:i32)
        n253 = xnode ("Saturation Subtract3")("x"=w575, "y"=w574) -> ("x-y"=w573:i32)
      }
    }
    "Acceleration (Counts/Interval) 2" <- w363
    "Velocity (Counts/Interval) 2" <- w362
    n254 = case shown="True" w351 {
      tunnel: w350 -> [_ w518]
      tunnel: w356 -> [w515 w522]
      tunnel: [w517 w521] -> w355
      tunnel: w358 -> [w517 w520]
      tunnel: [w516 w519] -> w354
      tunnel: w357 -> [w516 _]
      tunnel: [w515 w518] -> w353
      frame False {
      }
      frame True {
        n255 = xnode ("Saturation Subtract")("x"=w518, "y"=w522) -> ("x-y"=w521:i32)
        n256 = xnode ("Saturation Subtract3")("x"=w521, "y"=w520) -> ("x-y"=w519:i32)
      }
    }
    "Acceleration (Counts/Interval) 3" <- w354
    "Velocity (Counts/Interval) 3" <- w355
    n257 = case shown="True" w339 {
      tunnel: w334 -> [_ w464]
      tunnel: w342 -> [w461 w468]
      tunnel: [w463 w467] -> w335
      tunnel: w344 -> [w463 w466]
      tunnel: [w462 w465] -> w336
      tunnel: w343 -> [w462 _]
      tunnel: [w461 w464] -> w337
      frame False {
      }
      frame True {
        n258 = xnode ("Saturation Subtract")("x"=w464, "y"=w468) -> ("x-y"=w467:i32)
        n259 = xnode ("Saturation Subtract3")("x"=w467, "y"=w466) -> ("x-y"=w465:i32)
      }
    }
    "Acceleration (Counts/Interval) 4" <- w336
    "Velocity (Counts/Interval) 4" <- w335
  }
  n260 = node-c288() -> (w10:T2)  [unwired: 1 in]
  n261 = node-c288() -> (w12:T2)  [unwired: 1 in]
  n262 = timed-loop {
    timing: w10 -> [_]
    timing-out: [_] -> w9
    stop <- _ stop-if-true
    # "ENABLE MOTOR"
    n263 = xnode "FPGA I/O Node"("ConnectorB/DIO13"="En1", "ConnectorB/DIO14"="En2", "ConnectorB/DIO15"="En3", "ConnectorA/DIO13"="En4", "ConnectorA/DIO14"="En5", "ConnectorA/DIO15"="En6", "ConnectorC/DIO0"="En7", "ConnectorC/DIO1"="En8") -> ()  [unwired: 8 in, 8 out]
  }
  n264 = timed-loop {
    timing: w12 -> [_]
    timing-out: [_] -> w11
    stop <- _ stop-if-true
    # "Relay"
    n265 = xnode "FPGA I/O Node"("ConnectorB/DIO3"="Relay Motor 1", "ConnectorB/DIO4"="Relay motor 2", "ConnectorB/DIO5"="Relay motor 3", "ConnectorB/DIO6"="Relay motor 4", "ConnectorB/DIO7"="Relay kebocoran") -> ()  [unwired: 5 in, 5 out]
  }
  n266 = node-c288(w9) -> ()
  n267 = node-c288(w11) -> ()
  n268 = node-c288(w17) -> ()
  n269 = node-c288(w13) -> ()
